vi "题目4.vi"() -> ()   [LabVIEW 2017]
uses:
  <vilib>/Analysis/2dsp.llb/Real FFT.vi
  <vilib>/measure/NI_MABase.lvlib
  <vilib>/Analysis/NI_AALPro.lvlib
panel:
  out "频域信号":dbl[](graph)
  out "时域信号":dbl[](graph)
  in  "amplitude 3":dbl=1.0 caption="幅值" format="%0.2p"
  in  "frequency 3":dbl=10.0 caption="频率" format="%0.2p"
  in  "amplitude 2":dbl=1.0 caption="幅值" format="%0.2p"
  in  "frequency 2":dbl=10.0 caption="频率" format="%0.2p"
  in  "sampling info":cluster{"Fs":dbl, "#s":dbl}={"Fs"=1000.0, "#s"=1000.0} caption="采样信息" {"Fs" format="%.2p"}
  in  "amplitude":dbl=1.0 caption="幅值" format="%0.2p"
  in  "frequency":dbl=10.0 caption="频率" format="%0.2p"
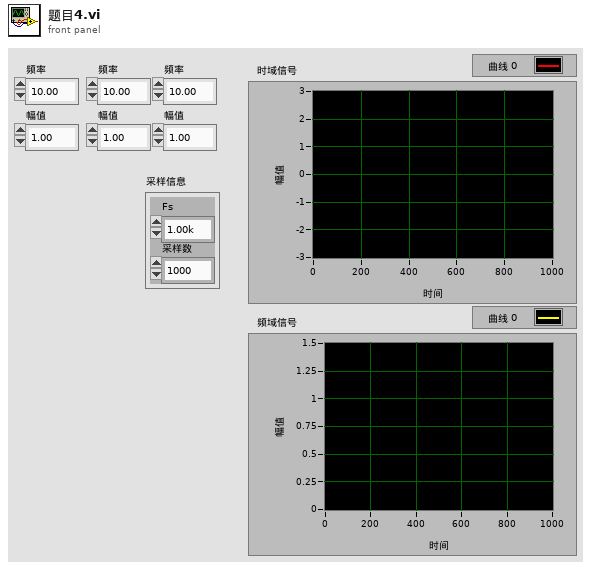
[diagram p1: front panel]
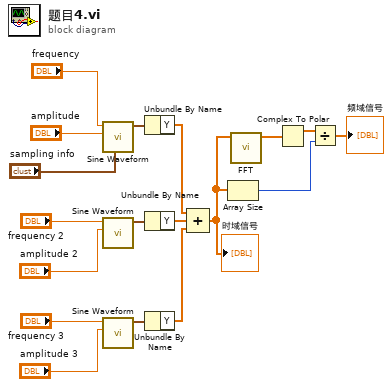
[diagram p0: block diagram]
diagram:
  n1 = call <vilib>:"Sine Waveform.vi"("sampling info"="sampling info", "amplitude"="amplitude", "frequency"="frequency") -> ("signal out"=w11:waveform(dbl))  [unwired: 7 in, 1 out]
  n2 = call <vilib>:"Sine Waveform.vi"("amplitude"="amplitude 2", "frequency"="frequency 2") -> ("signal out"=w10:waveform(dbl))  [unwired: 8 in, 1 out]
  n3 = call <vilib>:"Sine Waveform.vi"("amplitude"="amplitude 3", "frequency"="frequency 3") -> ("signal out"=w9:waveform(dbl))  [unwired: 8 in, 1 out]
  n4 = Unbundle By Name(w11) -> ("Y"=w8:dbl[])
  n5 = Unbundle By Name(w10) -> ("Y"=w7:dbl[])
  n6 = Unbundle By Name(w9) -> ("Y"=w6:dbl[])
  n7 = Compound Arithmetic op=ADD ("复合运算")(w8, w7, w6) -> (w5:dbl[])
  "时域信号" <- w5
  n8 = Array Size(array=w5) -> (size(s)=w2:i32)
  n9 = call-poly <vilib>:"FFT.vi"("X"=w5) -> ("FFT {X}"=w4:cdb[])  [unwired: 9 in, 1 out]
  n10 = Complex To Polar(r * e^(i*theta)=w4) -> (r=w3:dbl[])  [unwired: 1 out]
  n11 = Divide(x=w3, y=w2) -> (x/y=→"频域信号":dbl[])
